vi "Prober_InitObject.vi"(8 "error in (no error)":errorcluster, 10 "Prober Configuration":variant, 11 "AlessiRel6100 in":refnum<class "AlessiRel6100.lvclass">) -> (0 "error out":errorcluster, 3 "AlessiRel6100 out":refnum<class "AlessiRel6100.lvclass">)   [LabVIEW 2019, in "AlessiRel6100.lvclass"]
uses:
  AlessiRel6100.lvclass
  Alessi.vi
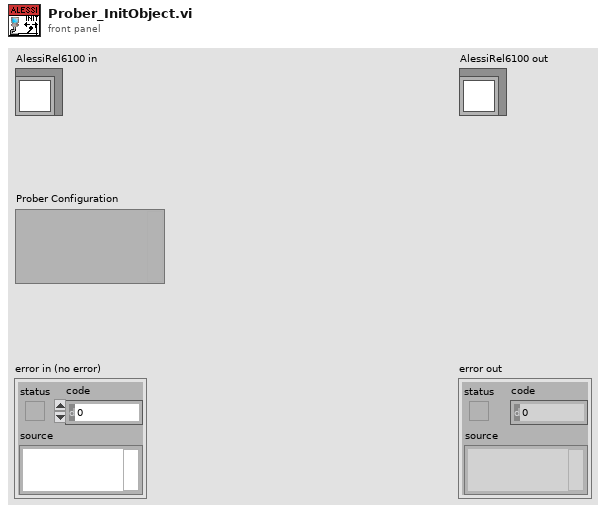
[diagram p1: front panel]
types:
  T1 = cluster{"Device ID Probe Station":u32, "Ref No.":u32, "Touchdown method":enum16{"no feedback", "Arduino edgesense"}, "Arduino Edgesense params":cluster{"touchdown height [µm]":i32, "search band [µm]":u32, "speed [µm/step]":u32, "overdrive [µm]":u32}}
  T2 = cluster{"touchdown height [µm]":i32, "search band [µm]":u32, "speed [µm/step]":u32, "overdrive [µm]":u32}
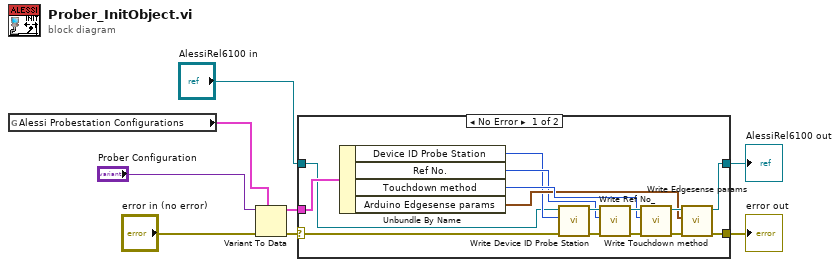
[diagram p0: block diagram]
diagram:
  n1 = global read "Alessi.vi" "Alessi Probestation Configurations"() -> (w2:T1)
  n2 = Variant To Data(error in="error in (no error)", type=w2, Variant="Prober Configuration") -> (data=w1:T1, error out=w4:errorcluster)
  n3 = case shown="No Error" w4 {
    selector: w4 -> [w12 w25]
    tunnel: "AlessiRel6100 in" -> [w9 w24]
    tunnel: [w10 w25] -> w7
    tunnel: [w11 w24] -> w6
    tunnel: w1 -> [w17 _]
    frame No Error {
      n4 = Unbundle By Name(w17) -> ("Device ID Probe Station"=w13:u32, "Ref No."=w14:u32, "Touchdown method"=w16:enum16{"no feedback", "Arduino edgesense"}, "Arduino Edgesense params"=w15:T2)
      n5 = call-dynamic "Write Device ID Probe Station.vi"("error in (no error)"=w12, "Device ID Probe Station"=w13, "AlessiRel6100 in"=w9) -> ("error out"=w22:errorcluster, "AlessiRel6100 out"=w23:refnum<class "AlessiRel6100.lvclass">)  [unwired: 7 in]
      n6 = call-dynamic "Write Ref No_.vi"("error in (no error)"=w22, "Ref No."=w14, "AlessiRel6100 in"=w23) -> ("error out"=w18:errorcluster, "AlessiRel6100 out"=w19:refnum<class "AlessiRel6100.lvclass">)  [unwired: 7 in]
      n7 = call-dynamic "Write Touchdown method.vi"("error in (no error)"=w18, "Touchdown method"=w16, "AlessiRel6100 in"=w19) -> ("error out"=w20:errorcluster, "AlessiRel6100 out"=w21:refnum<class "AlessiRel6100.lvclass">)  [unwired: 7 in]
      n8 = call-dynamic "Write Edgesense params.vi"("error in (no error)"=w20, "Edgesense params"=w15, "AlessiRel6100 in"=w21) -> ("error out"=w10:errorcluster, "AlessiRel6100 out"=w11:refnum<class "AlessiRel6100.lvclass">)  [unwired: 7 in]
    }
    frame Error {
    }
  }
  "error out" <- w7
  "AlessiRel6100 out" <- w6
